vi "TS_RST_SOURCE - Type.vi"(8 "error in (no error)":errorcluster) -> (0 "error out":errorcluster, 3 "TS_RST_SOURCE_VALUE":i32)   [LabVIEW 2015]
doc: "<b>Buffer policy settings can be only unsafe in xiAPI LabVIEW library</b>\nUNSAFE : User gets pointer to internally allocated circle buffer and data may be overwritten by device.\nSAFE : Data from device will be copied to user allocated buffer or xiApi allocated memory."
uses:
  C:/GIT/Cameras3.x/Integrations/Labview/xiLib/xiLIB_32bit/xiLIB/xiCamLib/API/x86/xiApi.NET.dll
  xiLIB_32bit/xiLIB/xiCamLib/API/x86/xiApi.NET.dll
  TS_RST_SOURCE.ctl
panel:
  in  "TS_RST_SOURCE":T1
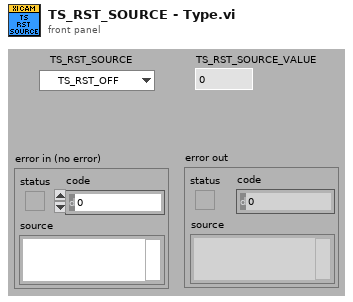
[diagram p1: front panel]
types:
  T1 = typedef "TS_RST_SOURCE.ctl" = enum16{"TS_RST_OFF", "TS_RST_SRC_GPI_1", "TS_RST_SRC_GPI_2", "TS_RST_SRC_GPI_3", "TS_RST_SRC_GPI_4", "TS_RST_SRC_GPI_1_INV", "TS_RST_SRC_GPI_2_INV", "TS_RST_SRC_GPI_3_INV", "TS_RST_SRC_GPI_4_INV", "TS_RST_SRC_GPO_1", "TS_RST_SRC_GPO_2", "TS_RST_SRC_GPO_3", "TS_RST_SRC_GPO_4", "TS_RST_SRC_GPO_1_INV", "TS_RST_SRC_GPO_2_INV", "TS_RST_SRC_GPO_3_INV", "TS_RST_SRC_GPO_4_INV", "TS_RST_SRC_TRIGGER", "TS_RST_SRC_TRIGGER_INV", "TS_RST_SRC_SW", "TS_RST_SRC_EXPACTIVE", "TS_RST_SRC_EXPACTIVE_INV", "TS_RST_SRC_FVAL", "TS_RST_SRC_FVAL_INV"}
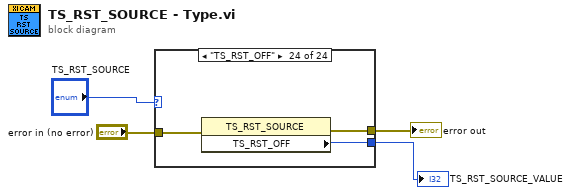
[diagram p0: block diagram]
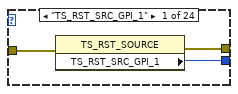
[diagram p2: hidden frame]
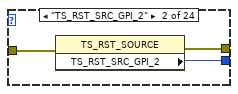
[diagram p3: hidden frame]
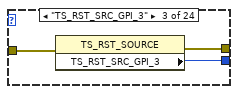
[diagram p4: hidden frame]
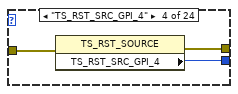
[diagram p5: hidden frame]
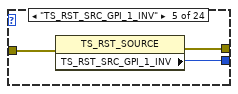
[diagram p6: hidden frame]
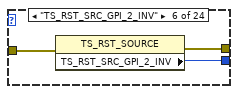
[diagram p7: hidden frame]
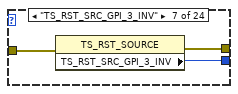
[diagram p8: hidden frame]
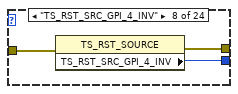
[diagram p9: hidden frame]
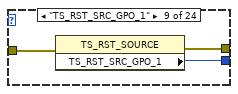
[diagram p10: hidden frame]
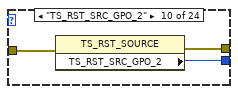
[diagram p11: hidden frame]
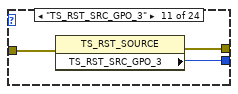
[diagram p12: hidden frame]
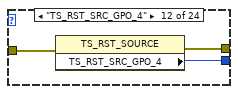
[diagram p13: hidden frame]
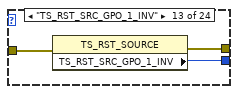
[diagram p14: hidden frame]
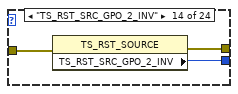
[diagram p15: hidden frame]
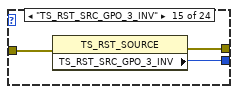
[diagram p16: hidden frame]
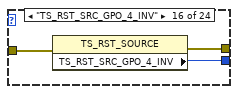
[diagram p17: hidden frame]
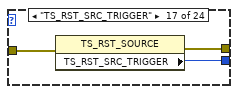
[diagram p18: hidden frame]
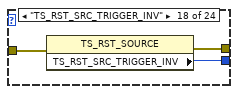
[diagram p19: hidden frame]
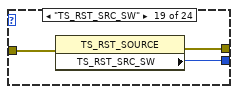
[diagram p20: hidden frame]
diagram:
  n1 = case shown="\"TS_RST_OFF\"" "TS_RST_SOURCE" {
    tunnel: "error in (no error)" -> [w7 w10 w13 w16 w19 w22 w25 w28 w31 w34 w37 w40 w43 w46 w49 w52 w55 w58 w61 w64 w67 w70 w73 w76]
    tunnel: [w6 w9 w12 w15 w18 w21 w24 w27 w30 w33 w36 w39 w42 w45 w48 w51 w54 w57 w60 w63 w66 w69 w72 w75] -> w3
    tunnel: [w5 w8 w11 w14 w17 w20 w23 w26 w29 w32 w35 w38 w41 w44 w47 w50 w53 w56 w59 w62 w65 w68 w71 w74] -> w2
    frame "TS_RST_SRC_GPI_1" {
      n2 = property class="TS_RST_SOURCE"(error in=w7) -> (error out=w6:errorcluster, "TS_RST_SRC_GPI_1"=w5:i32)  [unwired: 1 in, 1 out]
    }
    frame "TS_RST_SRC_GPI_2" {
      n3 = property class="TS_RST_SOURCE"(error in=w10) -> (error out=w9:errorcluster, "TS_RST_SRC_GPI_2"=w8:i32)  [unwired: 1 in, 1 out]
    }
    frame "TS_RST_SRC_GPI_3" {
      n4 = property class="TS_RST_SOURCE"(error in=w13) -> (error out=w12:errorcluster, "TS_RST_SRC_GPI_3"=w11:i32)  [unwired: 1 in, 1 out]
    }
    frame "TS_RST_SRC_GPI_4" {
      n5 = property class="TS_RST_SOURCE"(error in=w16) -> (error out=w15:errorcluster, "TS_RST_SRC_GPI_4"=w14:i32)  [unwired: 1 in, 1 out]
    }
    frame "TS_RST_SRC_GPI_1_INV" {
      n6 = property class="TS_RST_SOURCE"(error in=w19) -> (error out=w18:errorcluster, "TS_RST_SRC_GPI_1_INV"=w17:i32)  [unwired: 1 in, 1 out]
    }
    frame "TS_RST_SRC_GPI_2_INV" {
      n7 = property class="TS_RST_SOURCE"(error in=w22) -> (error out=w21:errorcluster, "TS_RST_SRC_GPI_2_INV"=w20:i32)  [unwired: 1 in, 1 out]
    }
    frame "TS_RST_SRC_GPI_3_INV" {
      n8 = property class="TS_RST_SOURCE"(error in=w25) -> (error out=w24:errorcluster, "TS_RST_SRC_GPI_3_INV"=w23:i32)  [unwired: 1 in, 1 out]
    }
    frame "TS_RST_SRC_GPI_4_INV" {
      n9 = property class="TS_RST_SOURCE"(error in=w28) -> (error out=w27:errorcluster, "TS_RST_SRC_GPI_4_INV"=w26:i32)  [unwired: 1 in, 1 out]
    }
    frame "TS_RST_SRC_GPO_1" {
      n10 = property class="TS_RST_SOURCE"(error in=w31) -> (error out=w30:errorcluster, "TS_RST_SRC_GPO_1"=w29:i32)  [unwired: 1 in, 1 out]
    }
    frame "TS_RST_SRC_GPO_2" {
      n11 = property class="TS_RST_SOURCE"(error in=w34) -> (error out=w33:errorcluster, "TS_RST_SRC_GPO_2"=w32:i32)  [unwired: 1 in, 1 out]
    }
    frame "TS_RST_SRC_GPO_3" {
      n12 = property class="TS_RST_SOURCE"(error in=w37) -> (error out=w36:errorcluster, "TS_RST_SRC_GPO_3"=w35:i32)  [unwired: 1 in, 1 out]
    }
    frame "TS_RST_SRC_GPO_4" {
      n13 = property class="TS_RST_SOURCE"(error in=w40) -> (error out=w39:errorcluster, "TS_RST_SRC_GPO_4"=w38:i32)  [unwired: 1 in, 1 out]
    }
    frame "TS_RST_SRC_GPO_1_INV" {
      n14 = property class="TS_RST_SOURCE"(error in=w43) -> (error out=w42:errorcluster, "TS_RST_SRC_GPO_1_INV"=w41:i32)  [unwired: 1 in, 1 out]
    }
    frame "TS_RST_SRC_GPO_2_INV" {
      n15 = property class="TS_RST_SOURCE"(error in=w46) -> (error out=w45:errorcluster, "TS_RST_SRC_GPO_2_INV"=w44:i32)  [unwired: 1 in, 1 out]
    }
    frame "TS_RST_SRC_GPO_3_INV" {
      n16 = property class="TS_RST_SOURCE"(error in=w49) -> (error out=w48:errorcluster, "TS_RST_SRC_GPO_3_INV"=w47:i32)  [unwired: 1 in, 1 out]
    }
    frame "TS_RST_SRC_GPO_4_INV" {
      n17 = property class="TS_RST_SOURCE"(error in=w52) -> (error out=w51:errorcluster, "TS_RST_SRC_GPO_4_INV"=w50:i32)  [unwired: 1 in, 1 out]
    }
    frame "TS_RST_SRC_TRIGGER" {
      n18 = property class="TS_RST_SOURCE"(error in=w55) -> (error out=w54:errorcluster, "TS_RST_SRC_TRIGGER"=w53:i32)  [unwired: 1 in, 1 out]
    }
    frame "TS_RST_SRC_TRIGGER_INV" {
      n19 = property class="TS_RST_SOURCE"(error in=w58) -> (error out=w57:errorcluster, "TS_RST_SRC_TRIGGER_INV"=w56:i32)  [unwired: 1 in, 1 out]
    }
    frame "TS_RST_SRC_SW" {
      n20 = property class="TS_RST_SOURCE"(error in=w61) -> (error out=w60:errorcluster, "TS_RST_SRC_SW"=w59:i32)  [unwired: 1 in, 1 out]
    }
    frame "TS_RST_SRC_EXPACTIVE" {
      n21 = property class="TS_RST_SOURCE"(error in=w64) -> (error out=w63:errorcluster, "TS_RST_SRC_EXPACTIVE"=w62:i32)  [unwired: 1 in, 1 out]
    }
    frame "TS_RST_SRC_EXPACTIVE_INV" {
      n22 = property class="TS_RST_SOURCE"(error in=w67) -> (error out=w66:errorcluster, "TS_RST_SRC_EXPACTIVE_INV"=w65:i32)  [unwired: 1 in, 1 out]
    }
    frame "TS_RST_SRC_FVAL" {
      n23 = property class="TS_RST_SOURCE"(error in=w70) -> (error out=w69:errorcluster, "TS_RST_SRC_FVAL"=w68:i32)  [unwired: 1 in, 1 out]
    }
    frame "TS_RST_SRC_FVAL_INV" {
      n24 = property class="TS_RST_SOURCE"(error in=w73) -> (error out=w72:errorcluster, "TS_RST_SRC_FVAL_INV"=w71:i32)  [unwired: 1 in, 1 out]
    }
    frame "TS_RST_OFF" {
      n25 = property class="TS_RST_SOURCE"(error in=w76) -> (error out=w75:errorcluster, "TS_RST_OFF"=w74:i32)  [unwired: 1 in, 1 out]
    }
  }
  "error out" <- w3
  "TS_RST_SOURCE_VALUE" <- w2
